vi "Ini key read (DBL).vi"(7 "Section name":string, 8 "error in (no error)":errorcluster, 10 "Parameter names & setup":T2, 11 "Ini file refnum in":T1) -> (0 "error out":errorcluster, 2 "Value read/used":dbl[](array[numeric]), 3 "Ini file refnum out":T1)   [LabVIEW 2017]
uses:
  Typedefs/Ini file interface (DBL).ctl
  <vilib>/Utility/config.llb/Config Data RefNum.ctl
  <vilib>/Utility/config.llb/Read Key (Double).vi
  <vilib>/Utility/config.llb/Write Key (Double).vi
  <vilib>/Utility/config.llb/NI_LVConfig.lvlib
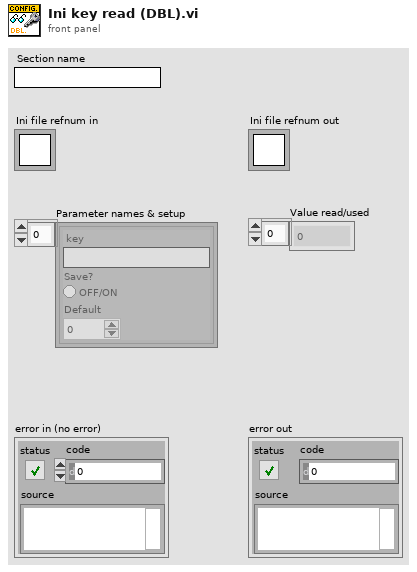
[diagram p1: front panel]
types:
  T1 = typedef "NI_LVConfig.lvlib/Config Data RefNum.ctl" = refnum<k1>
  T2 = typedef "Ini file interface (DBL).ctl" = cluster{"key":string, "Save?":bool, "Default":dbl}[]
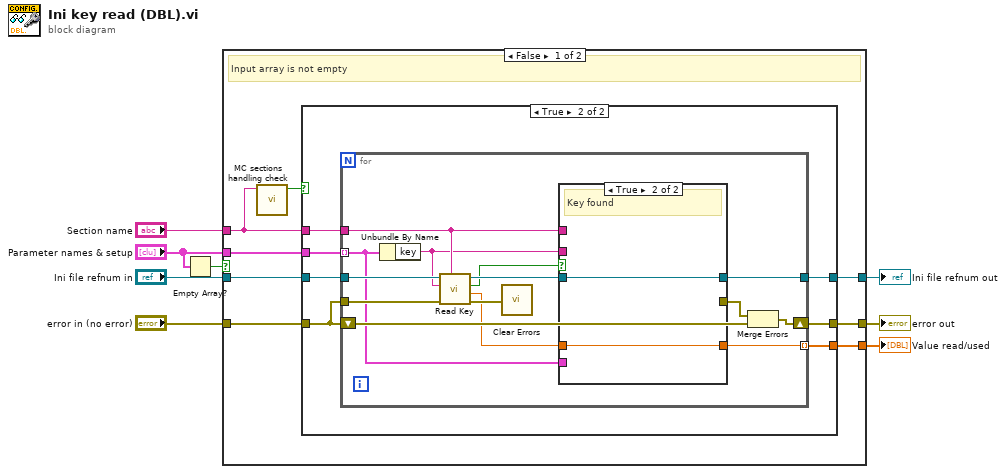
[diagram p0: block diagram]
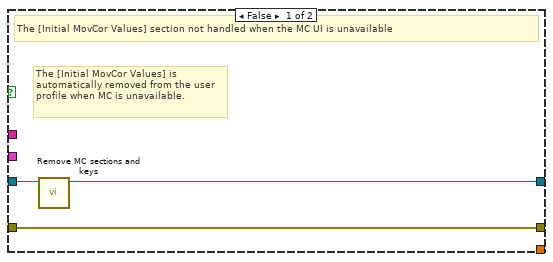
[diagram p2: hidden frame]
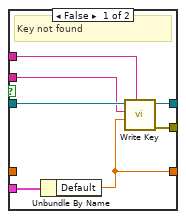
[diagram p3: hidden frame]
diagram:
  n1 = Empty Array?(array="Parameter names & setup") -> (empty?=w1:bool)
  n2 = case shown="False" w1 {
    tunnel: "Section name" -> [w10 _]
    tunnel: "Parameter names & setup" -> [w16 _]
    tunnel: [w15 _] -> w7
    tunnel: "error in (no error)" -> [w11 w50]
    tunnel: [w14 w50] -> w5
    tunnel: [w13 w51] -> w4
    tunnel: "Ini file refnum in" -> [w12 w51]
    frame False {
      # "Input array is not empty"
      n3 = call "MC sections handling check.vi"("Section name"=w10) -> ("Section is \"Initial MovCor Values\" AND MC is supported"=w9:bool)  [unwired: 10 in]
      n4 = case shown="True" w9 {
        tunnel: w16 -> [_ w26]
        tunnel: [_ w25] -> w15
        tunnel: [w18 w24] -> w14
        tunnel: [w17 w23] -> w13
        tunnel: w12 -> [w19 w22]
        tunnel: w11 -> [w18 w21]
        tunnel: w10 -> [_ w20]
        frame False {
          # "The [Initial MovCor Values] is automatically removed from the user profile when MC is unavailable."
          # "The [Initial MovCor Values] section not handled when the MC UI is unavailable"
          n5 = call "Remove MC sections and keys.vi"("User profile ref"=w19) -> ("User profile ref"=w17:T1)  [unwired: 10 in]
        }
        frame True {
          n6 = for {
            tunnel: w20 -> [w33]
            tunnel: w22 -> [w40]
            tunnel: w21 -> [w39]
            tunnel: [w36] -> w23
            shift-right: [w38] -> w24
            shift-left: w21 -> [w37]
            tunnel: w26 -> [w34] mode=indexing
            tunnel: [w35] -> w25 mode=indexing
            n7 = Unbundle By Name(w34) -> ("key"=w27:string)
            n8 = call-poly <vilib>:"Read Key.vi"("section"=w33, "error in (no error)"=w39, "key"=w27, "refnum"=w40) -> ("error out"=w32:errorcluster, "value"=w28:dbl, "found?"=w29:bool, "refnum out"=w31:T1)  [unwired: 4 in]
            n9 = call <vilib>:"Clear Errors.vi"("error in (no error)"=w32) -> ()  [unwired: 5 in, 2 out]
            n10 = case shown="True" w29 {
              tunnel: w31 -> [w47 w49]
              tunnel: [w46 w49] -> w36
              tunnel: [w45 _] -> w30
              tunnel: w33 -> [w44 _]
              tunnel: w27 -> [w43 _]
              tunnel: w28 -> [_ w48]
              tunnel: [w41 w48] -> w35
              tunnel: w34 -> [w42 _]
              frame False {
                # "Key not found"
                n11 = Unbundle By Name(w42) -> ("Default"=w41:dbl)
                n12 = call-poly <vilib>:"Write Key.vi"("section"=w44, "value"=w41, "key"=w43, "refnum"=w47) -> ("error out"=w45:errorcluster, "refnum out"=w46:T1)  [unwired: 5 in, 1 out]
              }
              frame True {
                # "Key found"
              }
            }
            n13 = Merge Errors(w30, w37) -> (w38:errorcluster)
          }
        }
      }
    }
    frame True {
      # "Input array is empty"
    }
  }
  "Value read/used" <- w7
  "error out" <- w5
  "Ini file refnum out" <- w4
